vi "extractNewValueFromEvent.vi"(8 "error in (no error)":errorcluster, 10 "channelName":string, 11 "ScriptListCompiler in":refnum<class "ScriptListCompiler.lvclass">) -> (0 "error out":errorcluster, 2 "newValue":string, 3 "ScriptListCompiler out":refnum<class "ScriptListCompiler.lvclass">)   [LabVIEW 2009, in "Compiler.lvlib" / "ScriptListCompiler.lvclass"]
uses:
  ScriptListCompiler.lvclass
  ScriptListCompiler.lvclass/ScriptListCompiler.ctl
  Scripting/ScriptingEvent/ScriptEventList/ScriptEventList.lvclass
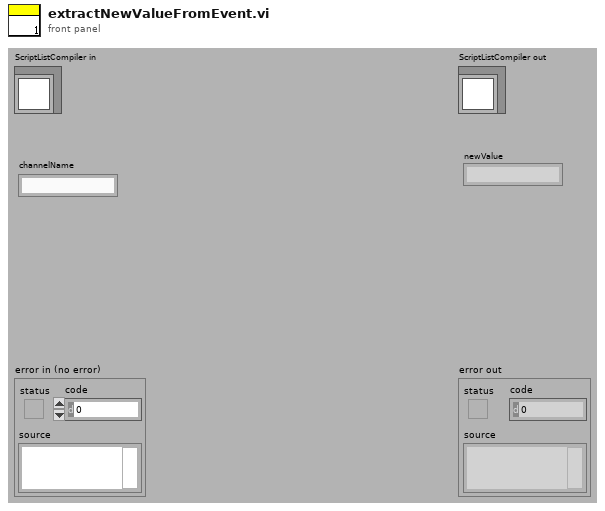
[diagram p1: front panel]
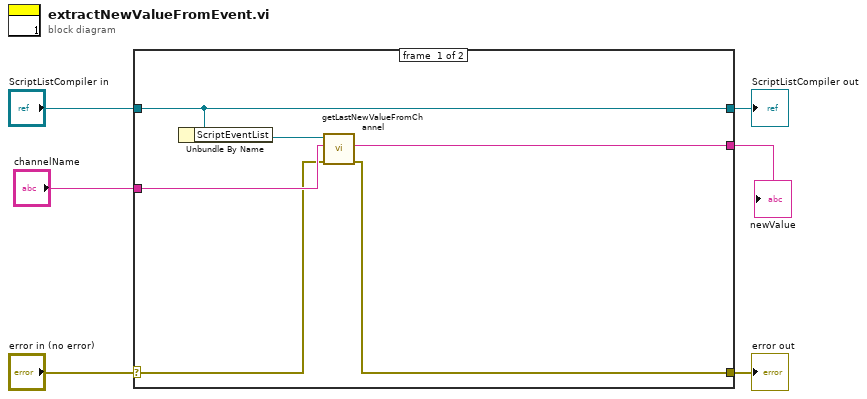
[diagram p0: block diagram]
diagram:
  n1 = case shown="No Error" "error in (no error)" {
    selector: "error in (no error)" -> [w9 w14]
    tunnel: [w8 w14] -> w5
    tunnel: [w12 w13] -> w3
    tunnel: "ScriptListCompiler in" -> [w12 w13]
    tunnel: "channelName" -> [w10 _]
    tunnel: [w7 _] -> w1
    frame #0 {
      n2 = Unbundle By Name(w12) -> ("ScriptEventList"=w11:refnum<class "ScriptEventList.lvclass">)
      n3 = call "getLastNewValueFromChannel.vi"("error in (no error)"=w9, "channelName"=w10, "ScriptEventList in"=w11) -> ("error out"=w8:errorcluster, "newValue"=w7:string)  [unwired: 6 in, 1 out]
    }
    frame #1 {
    }
  }
  "error out" <- w5
  "ScriptListCompiler out" <- w3
  "newValue" <- w1
